vi "Set ForceActuatorBoosterValveGainSettings.vi"(10 "ForceActuatorBoosterValveGainSettings":T1, 11 "Model in":refnum<class "Model.lvclass">) -> (3 "Model out":refnum<class "Model.lvclass">)   [LabVIEW 2016, in "Model.lvclass"]
uses:
  Model.lvclass
  Typedefs/ForceActuatorBoosterValveGainSettings.ctl
  Model.lvclass/Model.ctl
  Typedefs/FAMT Typedefs.lvlib
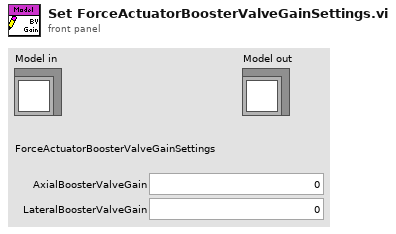
[diagram p1: front panel]
types:
  T1 = typedef "FAMT Typedefs.lvlib/ForceActuatorBoosterValveGainSettings.ctl" = cluster{"AxialBoosterValveGain":sgl, "LateralBoosterValveGain":sgl}
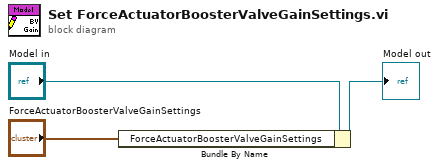
[diagram p0: block diagram]
diagram:
  n1 = Bundle By Name(cluster="Model in", "ForceActuatorBoosterValveGainSettings"="ForceActuatorBoosterValveGainSettings") -> (→"Model out":refnum<class "Model.lvclass">)
